vi "Mechanism-names.vi"(7 "Slot/filter  number":u16, 10 "Mechanism  number":u16, 11 "Mechanism type":u16(ring) items=["Filter wheels", "Focus"]) -> (1 "Selected wheel  filter names arr":string[](array[string]), 2 "Mech  names arr out":string[](array[string])=["FW-YJ", "FW-HK", "Slit-wheel", "FW-aux"], 3 "Mechanism name":string, 5 "Selected filter name":string)   [LabVIEW 2022 SP3]
panel:
  in  "Aux filter names":string[](array[string])=["0", "1", "2", "3", "4", "5", "6", "7"]
  in  "Slits names":string[](array[string])=["135", "blocked", "80", "open 1", "250", "open"]
  in  "HK filter names":string[](array[string])=["Grism", "blocked", "VPH", "open", "H", "K"]
  in  "YJ filter names":string[](array[string])=["Grism", "blocked", "VPH", "open", "J", "Y"]
  in  "Focus mechanisms":string[](array[string])=["Focus-YJ", "Focus-HK", "Focus-InSb"]
  in  "FW names":string[](array[string])=["FW-YJ", "FW-HK", "Slit-wheel", "FW-aux"]
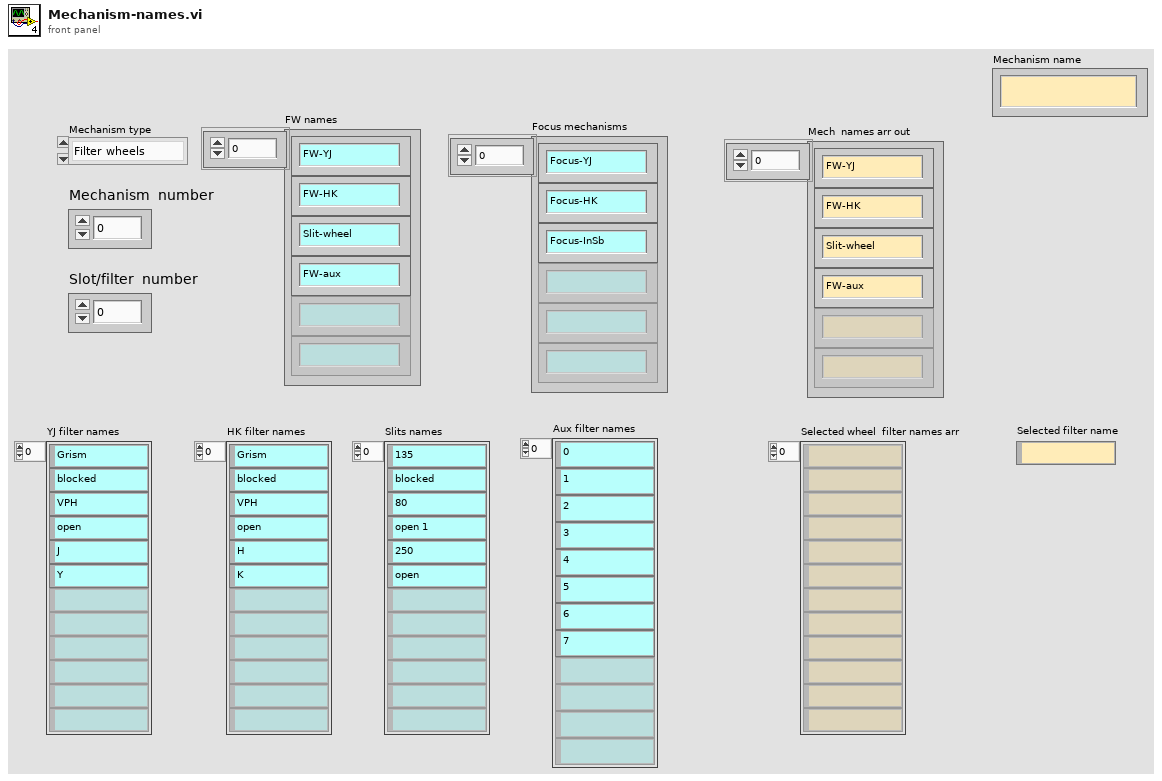
[diagram p1: front panel]
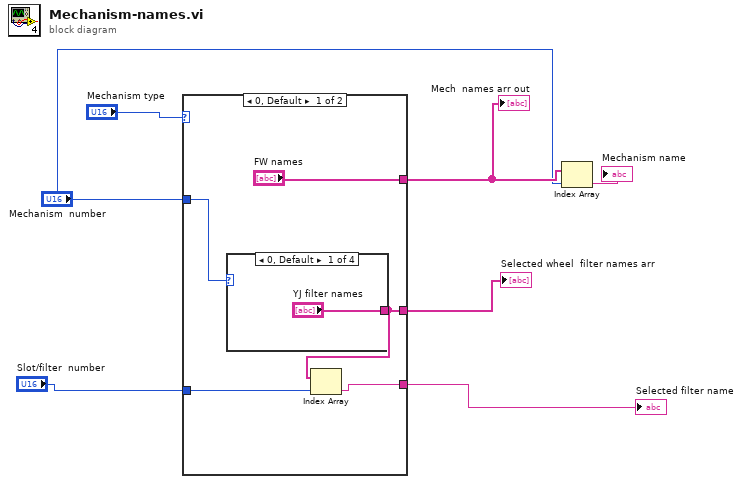
[diagram p0: block diagram]
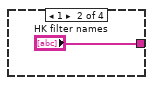
[diagram p2: hidden frame]
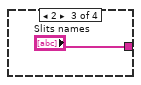
[diagram p3: hidden frame]
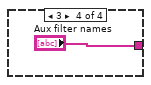
[diagram p4: hidden frame]
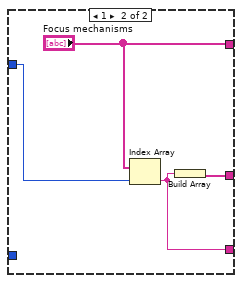
[diagram p5: hidden frame]
diagram:
  n1 = case shown="0, Default" "Mechanism type" {
    tunnel: ["FW names" "Focus mechanisms"] -> w5
    tunnel: "Mechanism  number" -> [w11 w20]
    tunnel: [w10 w18] -> w3
    tunnel: "Slot/filter  number" -> [w9 _]
    tunnel: [w8 w17] -> w1
    frame 0, Default {
      n2 = case shown="0, Default" w11 {
        tunnel: ["YJ filter names" "HK filter names" "Slits names" "Aux filter names"] -> w10
        frame 0, Default {
        }
        frame 1 {
        }
        frame 2 {
        }
        frame 3 {
        }
      }
      n3 = Index Array(array=w10, index=w9) -> (element=w8:string)
    }
    frame 1 {
      n4 = Index Array(array="Focus mechanisms", index=w20) -> (element=w17:string)
      n5 = Build Array(w17) -> (w18:string[])
    }
  }
  "Mech  names arr out" <- w5
  "Selected wheel  filter names arr" <- w3
  "Selected filter name" <- w1
  n6 = Index Array(array=w5, index="Mechanism  number") -> (element=→"Mechanism name":string)
